vi "main.vi"(8 "Error In":errorcluster, 9 "Simulation Module":bool[](array[boolean]), 10 "Application Path Cluster":T1, 11 "Software Name":string) -> (0 "Error Out":errorcluster)   [LabVIEW 2018]
uses:
  controls/pathCluster.ctl
  UI Module/src/controls/uiData.ctl
  controls/controllerData.ctl
  controls/openModbusConnectionCluster.ctl
  Simulation Module/src/controls/simulationData.ctl
  PLC Module/src/controls/plcData.ctl
  Barcode Scanner Module/src/controls/scanData.ctl
  Barcode Printer Module/src/controls/printData.ctl
  PLC Module/src/controls/plcUDE.ctl
  UI Module/src/controls/uiUDE.ctl
  Simulation Module/src/controls/Simulation UDE.ctl
  <vilib>/event_ctls.llb/usereventprio.ctl
  885446ab-6654-46eb-9afe-71431fbeab30.vi
  367c2bb0-f26a-4887-9fcf-0ea6fc163310.vi
  079b8fb7-678e-4098-9aed-ba415320bfda.vi
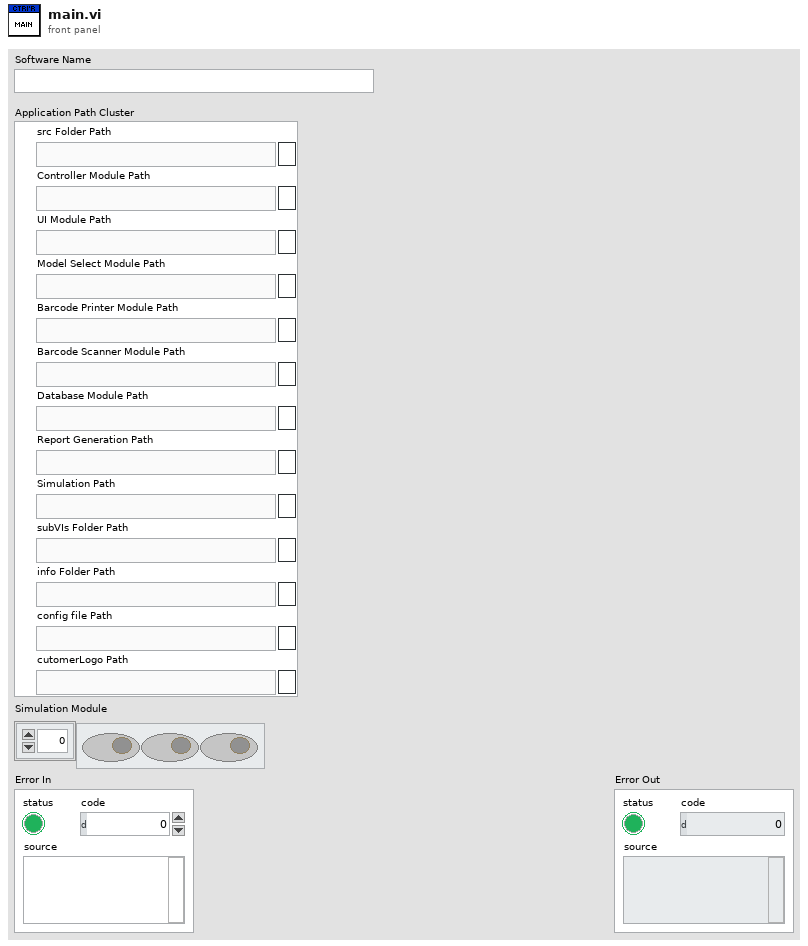
[diagram p1: front panel]
types:
  T1 = typedef "pathCluster.ctl" = cluster{"src Folder Path":path, "Controller Module Path":path, "UI Module Path":path, "Model Select Module Path":path, "Barcode Printer Module Path":path, "Barcode Scanner Module Path":path, "Database Module Path":path, "Report Generation Path":path, "Simulation Path":path, "subVIs Folder Path":path, "info Folder Path":path, "config file Path":path, "cutomerLogo Path":path}
  T2 = enum32{"Invalid", "Standard", "Closed", "Hidden", "Minimized", "Maximized"}
  T3 = enum32{"invalid app kind", "Development System", "Run Time System", "Student Edition", "Embedded LabVIEW", "Evaluation", "Custom"}
  T4 = typedef "plcUDE.ctl" = cluster{"Stop UDE":refnum<user-event>, "PLC UDE":refnum<user-event>}
  T5 = typedef "uiUDE.ctl" = cluster{"UI UDE":refnum<user-event>, "Stop UDE":refnum<user-event>}
  T6 = typedef "Simulation UDE.ctl" = cluster{"Stop UDE":refnum<user-event>, "Simulation Data":refnum<user-event>}
  T7 = typedef "plcData.ctl" = cluster{"IP Address":string, "Timeout":i32, "Port [502]":u16, "isSimulation?":bool, "Model Number":u16}
  T8 = typedef "uiData.ctl" = cluster{"Software Name":string, "UI Module Path":path}
  T9 = typedef "simulationData.ctl" = cluster{"Port [502]":u16, "Model Number":u16}
  T10 = typedef "usereventprio.ctl" = enum32{"high priority", "normal priority"}
  T11 = typedef "openModbusConnectionCluster.ctl" = cluster{"IP Address":string, "Timeout (ms)":i32, "Port (502)":u16}
  T12 = cluster{"Core":cluster{"Current VI Reference":refnum<vi>, "Close Panel on Exit?":bool}, "Software Name":string, "Application Path Cluster":T1, "Simulation Module":bool[], "Open Modbus Connection Cluster":T11, "PLC Data":T7, "Stop UDE":refnum<user-event>, "Simulation UDE":refnum<user-event>, "PLC UDE":refnum<user-event>, "Print Data":refnum<user-event>, "Scan UDE":refnum<user-event>, "Controller UDE":refnum<user-event>, "UI UDE":refnum<user-event>}
  T13 = cluster{"Current VI Reference":refnum<vi>, "Close Panel on Exit?":bool}
  T14 = typedef "scanData.ctl" = cluster{"Scan Button":bool}
  T15 = typedef "printData.ctl" = cluster{"Print Button":bool, "VISA resource name":refnum<visa-resource-name>, "Status?":bool, "Scan?":bool}
  T16 = typedef "controllerData.ctl" = cluster{"Sample":bool}
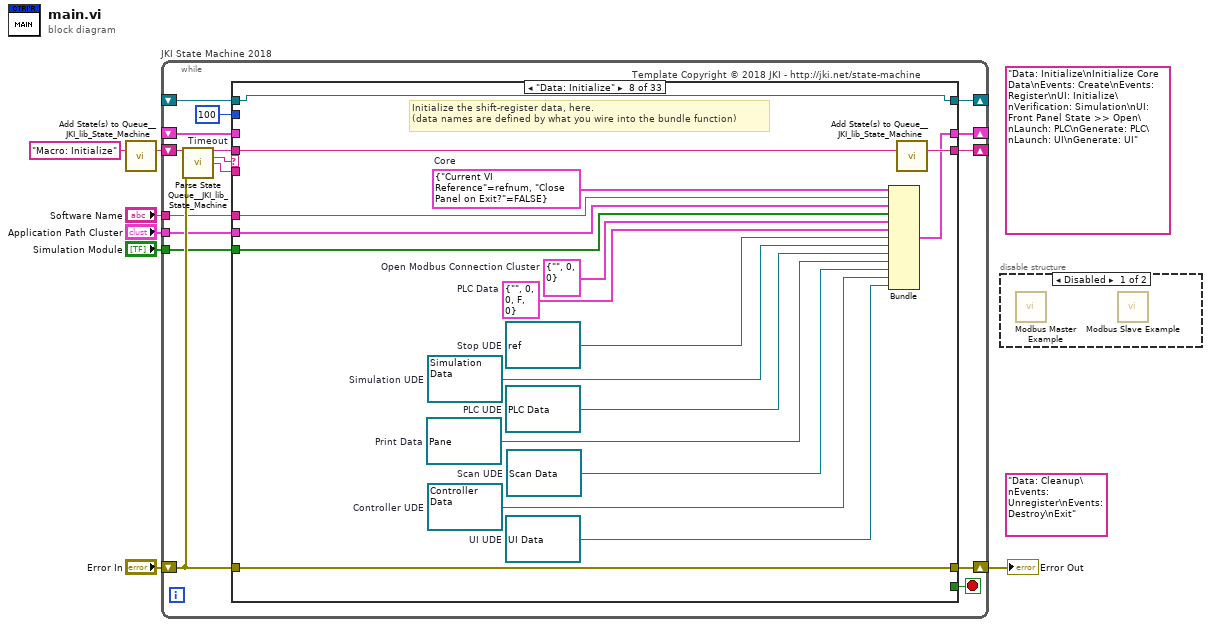
[diagram p0: block diagram]
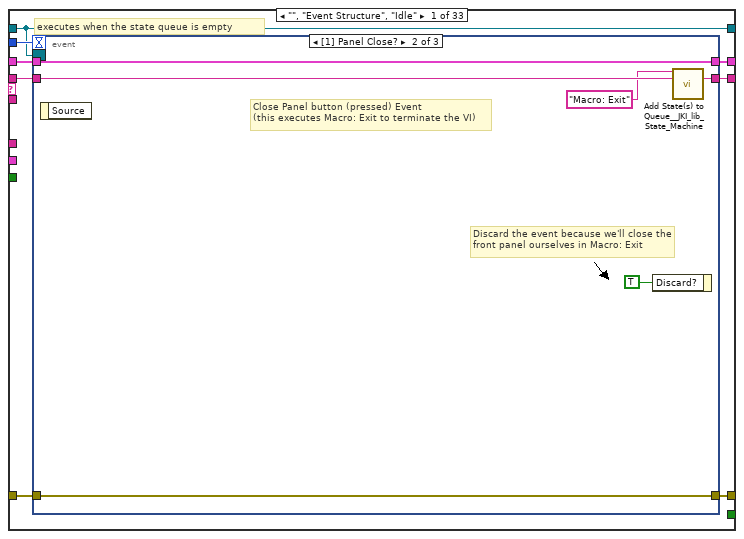
[diagram p3: hidden frame]
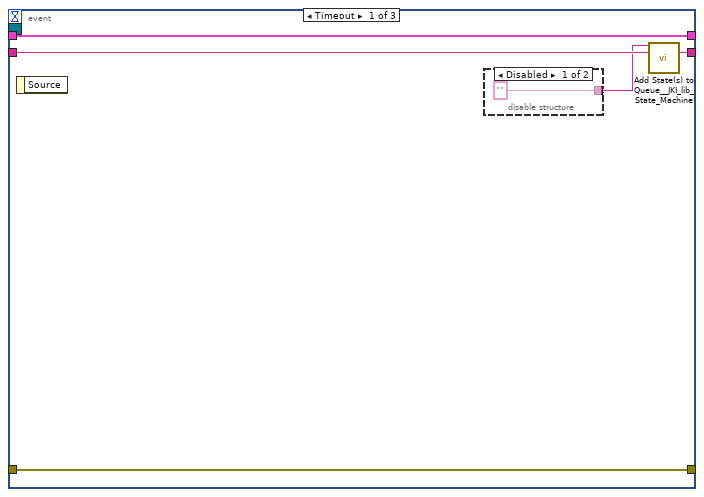
[diagram p4: hidden frame]
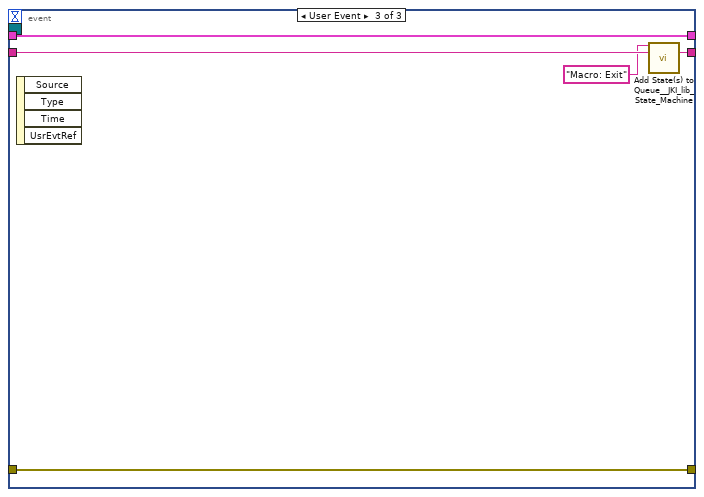
[diagram p6: hidden frame]
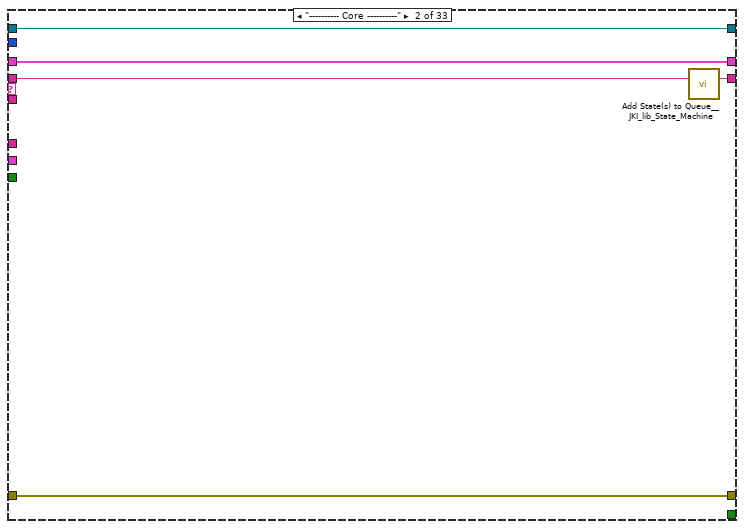
[diagram p7: hidden frame]
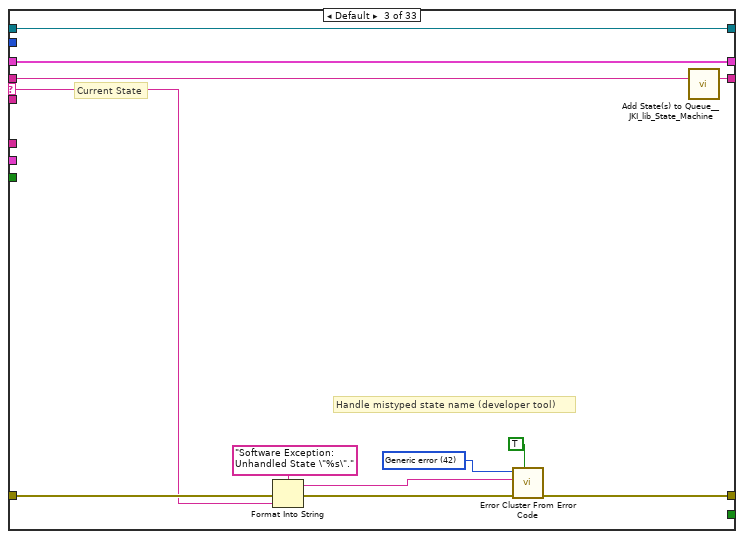
[diagram p8: hidden frame]
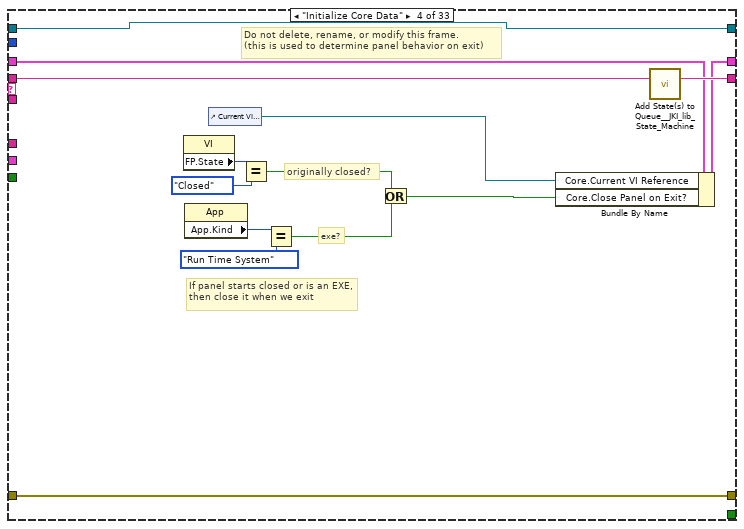
[diagram p9: hidden frame]
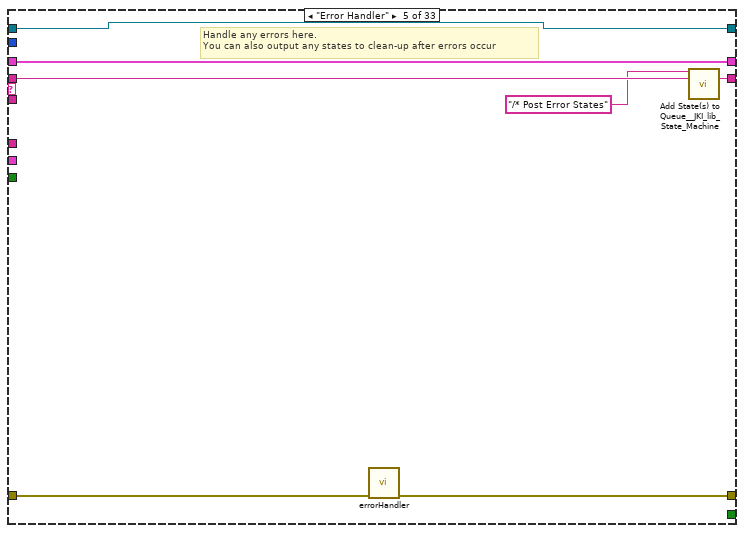
[diagram p10: hidden frame]
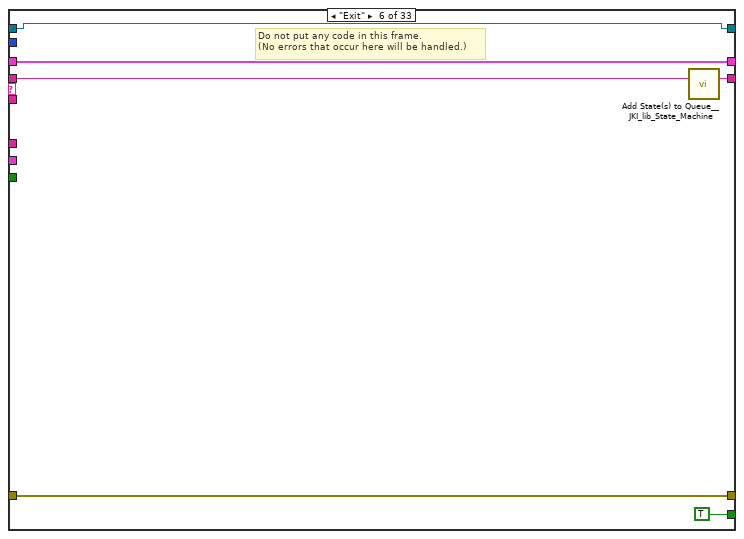
[diagram p11: hidden frame]
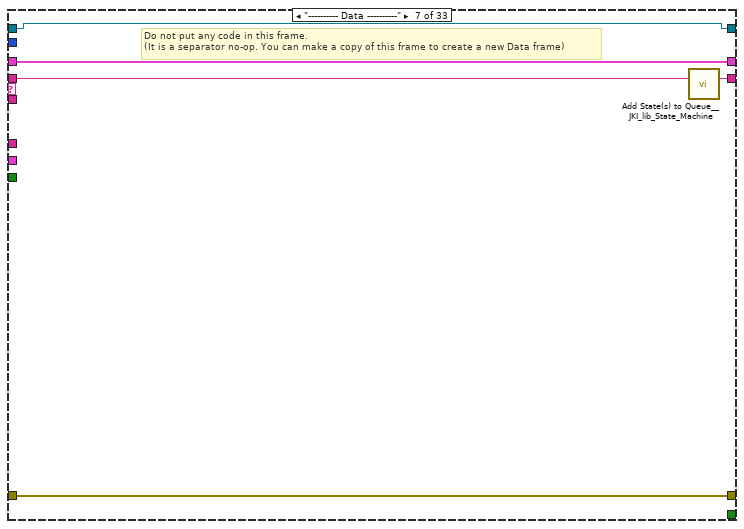
[diagram p12: hidden frame]
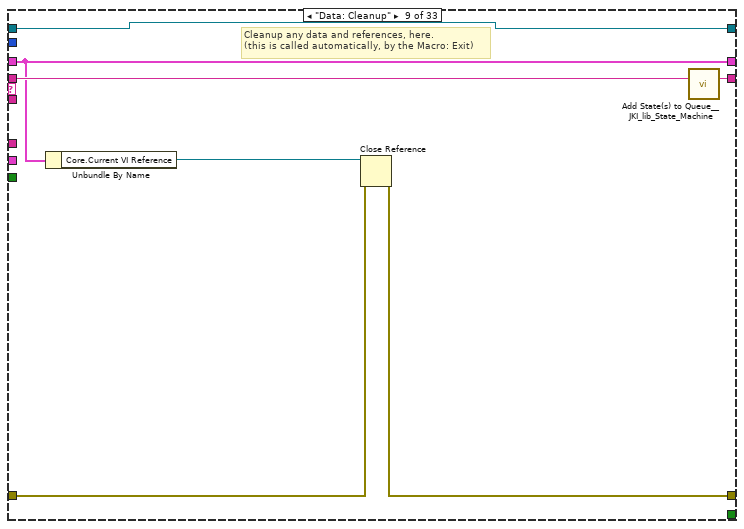
[diagram p13: hidden frame]
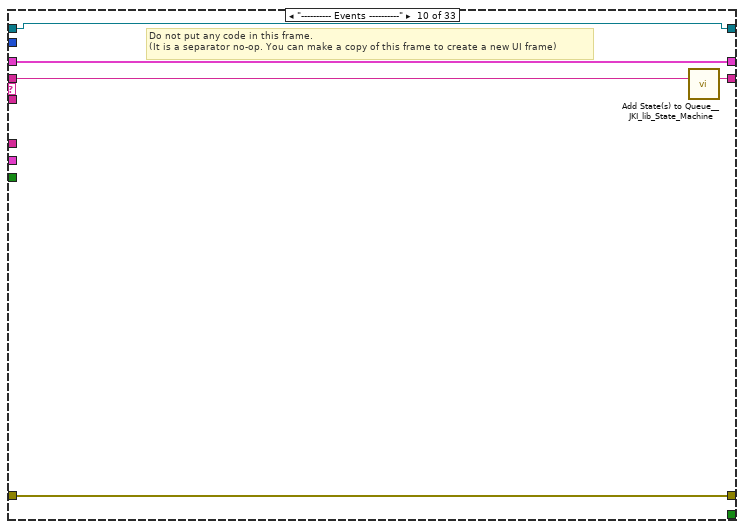
[diagram p14: hidden frame]
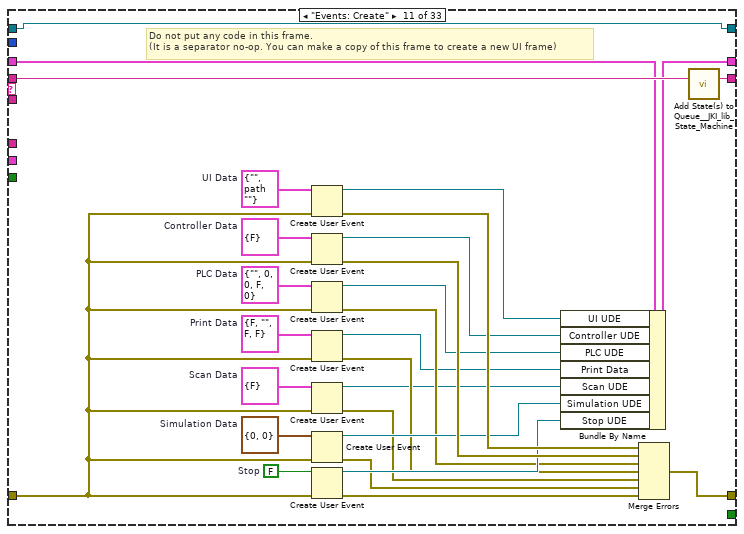
[diagram p15: hidden frame]
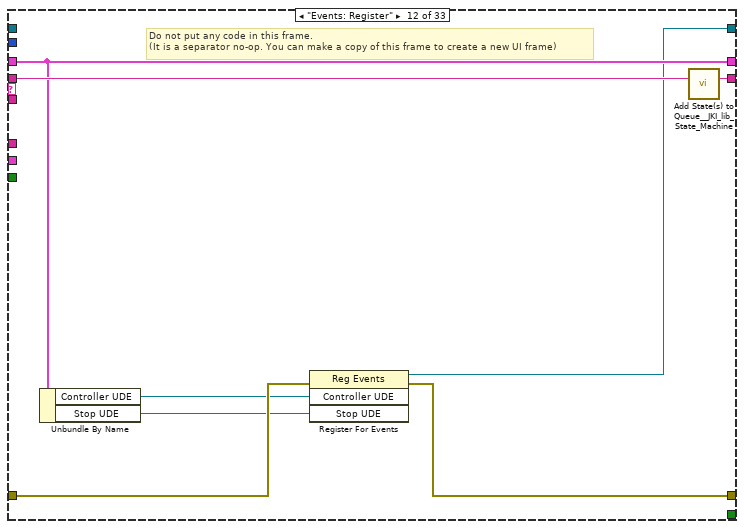
[diagram p16: hidden frame]
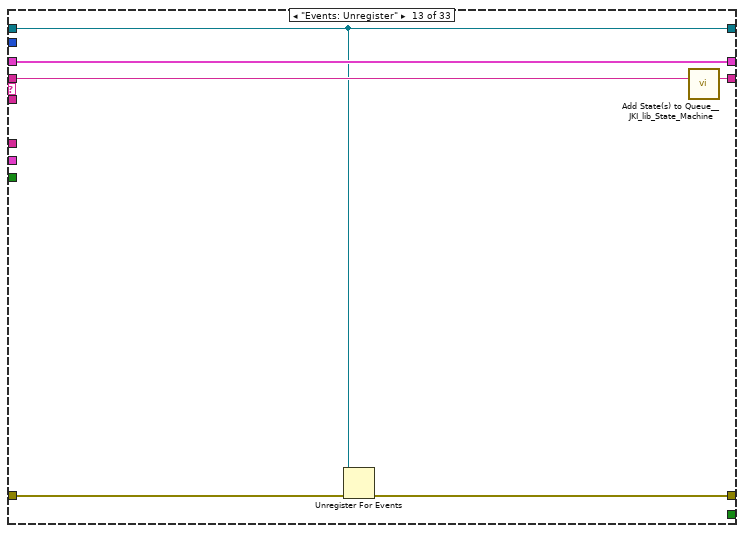
[diagram p17: hidden frame]
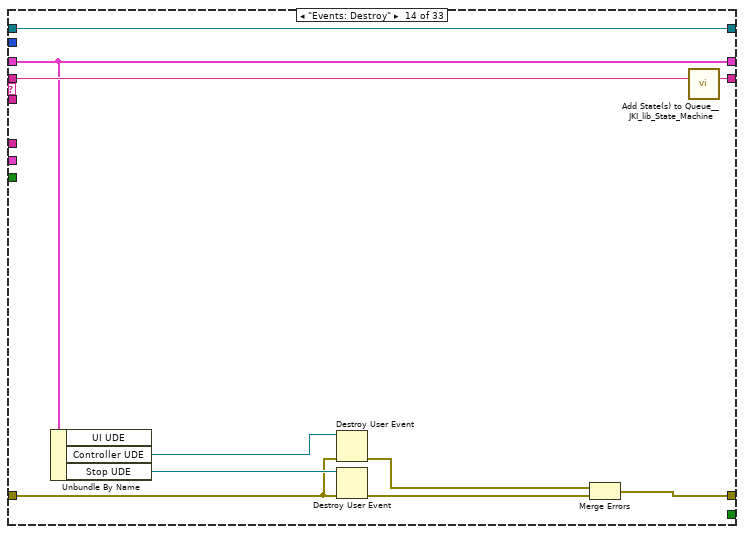
[diagram p18: hidden frame]
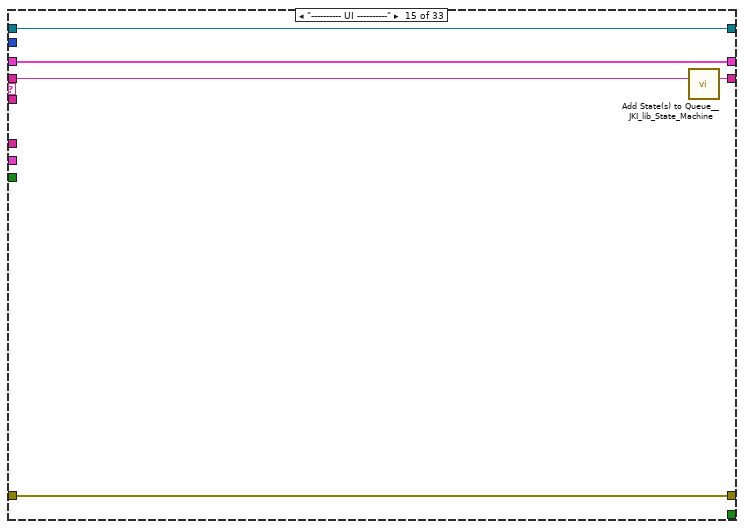
[diagram p19: hidden frame]
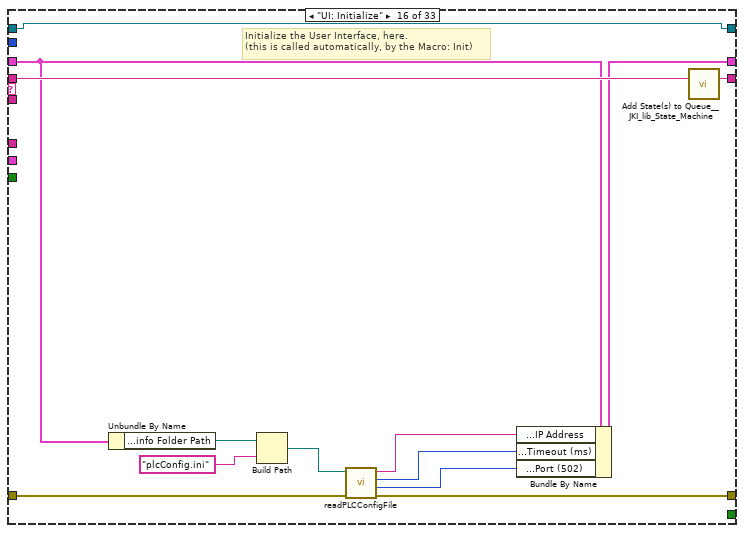
[diagram p20: hidden frame]
diagram:
  (unwired) "Data: Cleanup\nEvents: Unregister\nEvents: Destroy\nExit"
  (unwired) "Data: Initialize\nInitialize Core Data\nEvents: Create\nEvents: Register\nUI: Initialize\nVerification: Simulation\nUI: Front Panel State >> Open\nLaunch: PLC\nGenerate: PLC\nLaunch: UI\nGenerate: UI"
  n1 = call <vilib>:"Add State(s) to Queue__JKI_lib_State_Machine.vi"("State(s) in (\"\")"="Macro: Initialize") -> ("States Out"=w7:string)  [unwired: 14 in]
  n2 = while "JKI State Machine 2018" {
    shift-right: [w16] -> _
    shift-left: _ -> [w15]
    shift-right: [w19] -> w5
    shift-left: "Error In" -> [w13]
    shift-right: [w18] -> _
    shift-left: w7 -> [w20]
    shift-right: [w12] -> _
    shift-left: _ -> [w11]
    tunnel: "Simulation Module" -> [w10]
    tunnel: "Software Name" -> [w9]
    tunnel: "Application Path Cluster" -> [w8]
    stop <- w17 stop-if-true
    w14 = 100  # Timeout
    # "Template Copyright © 2018 JKI - http://jki.net/state-machine"
    n3 = call <vilib>:"Parse State Queue__JKI_lib_State_Machine.vi"("State Queue"=w20, "Error In (no error)"=w13) -> ("Remaining States"=w22:string, "Current State"=w23:string, "Arguments"=w21:string)  [unwired: 11 in]
    n4 = case shown="\"Data: Initialize\"" w23 {
      selector: w23 -> [_ _ w55 _ _ _ _ _ _ _ _ _ _ _ _ _ _ _ _ _ _ _ _ _ _ _ _ _ _ _ _ _ _]
      tunnel: w22 -> [w31 w53 w59 w79 w86 w92 w97 w115 w122 w127 w155 w163 w169 w179 w184 w197 w204 w216 w286 w292 w303 w308 w320 w332 w344 w349 w357 w364 w369 w386 w400 w412 w423]
      tunnel: w21 -> [_ _ _ _ _ _ _ _ _ _ _ _ _ _ _ _ w199 w210 _ _ _ _ _ _ _ _ _ _ _ _ _ _ _]
      tunnel: w15 -> [w29 w50 w57 w72 w84 w90 w94 _ w117 w124 w146 w161 w167 w175 w181 w191 w202 w212 w283 w289 w300 w305 w317 w329 w341 w346 w353 w361 w366 w374 w389 w406 w417]
      tunnel: [w28 w51 w61 w76 w80 w89 w95 w112 w118 w125 w151 w157 w165 w171 w182 w192 w200 w213 w284 w290 w301 w306 w310 w322 w334 w347 w355 w362 w367 w382 w396 w408 w419] -> w19
      tunnel: w13 -> [w27 w51 w60 w76 w81 w89 w95 w112 w119 w125 w128 w160 w166 w172 w182 w193 w201 w214 w284 w290 w301 w306 w316 w325 w339 w347 w355 w362 w367 w383 w397 w409 w420]
      tunnel: [w30 w52 w58 w78 w85 w91 w96 w114 w121 w126 w154 w162 w168 w178 w183 w196 w203 w215 w285 w291 w302 w307 w319 w331 w343 w348 w356 w363 w368 w385 w399 w411 w422] -> w18
      tunnel: [_ _ _ _ _ TRUE _ _ _ _ _ _ _ _ _ _ _ _ _ _ _ _ _ _ _ _ _ _ _ _ _ _ _] -> w17
      tunnel: [w26 w50 w57 w77 w84 w90 w94 w113 w117 w124 w142 w161 w167 w175 w181 w194 w202 w212 w283 w289 w300 w305 w317 w329 w341 w346 w353 w361 w366 w373 w388 w405 w416] -> w16
      tunnel: w14 -> [w25 _ _ _ _ _ _ _ _ _ _ _ _ _ _ _ _ _ _ _ _ _ _ _ _ _ _ _ _ _ _ _ _]
      tunnel: [w24 w49 w54 w66 w82 w87 w93 w107 w116 w123 w141 w156 w164 w177 w180 w195 w198 w209 w282 w287 w293 w304 w318 w330 w342 w345 w354 w360 w365 w384 w398 w410 w421] -> w12
      tunnel: w11 -> [w24 w49 w54 w66 w82 w87 w93 w107 w116 w123 w141 _ w164 w177 w180 w195 w198 w209 w282 w287 w293 w304 w318 w330 w342 w345 w354 w360 w365 w384 w398 w410 w421]
      tunnel: w10 -> [_ _ _ _ _ _ _ w105 _ _ _ _ _ _ _ _ _ _ _ _ _ _ _ _ _ _ _ _ _ _ _ _ _]
      tunnel: w9 -> [_ _ _ _ _ _ _ w104 _ _ _ _ _ _ _ _ _ _ _ _ _ _ _ _ _ _ _ _ _ _ _ _ _]
      tunnel: w8 -> [_ _ _ _ _ _ _ w103 _ _ _ _ _ _ _ _ _ _ _ _ _ _ _ _ _ _ _ _ _ _ _ _ _]
      frame "", "Event Structure", "Idle" {
        # "executes when the state queue is empty"
        n5 = event shown="[1] Panel Close?" {
          selector: w24 -> [_ _ _]
          dyn-events: _ -> [_ _ _]
          timeout: w25 -> [_ _ _]
          tunnel: w31 -> [w36 w43 w46]
          tunnel: [w35 w42 w47] -> w30
          tunnel: w29 -> [w33 w40 w48]
          tunnel: [w34 w41 w44] -> w28
          tunnel: w27 -> [w34 w41 w44]
          tunnel: [w33 w40 w48] -> w26
          event Timeout {
            n6 = event-data() -> ()  [unwired: 1 in, 1 out]
            n7 = disable-structure shown="Disabled" {
              disable-tunnel: ["" _] -> w32
              frame Disabled {
              }
              frame Enabled {
              }
            }
            n8 = call <vilib>:"Add State(s) to Queue__JKI_lib_State_Machine.vi"("State(s) in Front (\"\")"=w32, "State(s) in (\"\")"=w36) -> ("States Out"=w35:string)  [unwired: 13 in]
          }
          event Panel Close? {
            # "Discard the event because we'll close the front panel ourselves in Macro: Exit"
            # "Close Panel button (pressed) Event\n(this executes Macro: Exit to terminate the VI)"
            n9 = event-data() -> ()  [unwired: 1 in, 1 out]
            n10 = event-data("Discard?"=TRUE) -> ()  [unwired: 1 in, 1 out]
            n11 = call <vilib>:"Add State(s) to Queue__JKI_lib_State_Machine.vi"("State(s) in Front (\"\")"="Macro: Exit", "State(s) in (\"\")"=w43) -> ("States Out"=w42:string)  [unwired: 13 in]
          }
          event User Event {
            n12 = event-data() -> ()  [unwired: 1 in, 4 out]
            n13 = call <vilib>:"Add State(s) to Queue__JKI_lib_State_Machine.vi"("State(s) in Front (\"\")"="Macro: Exit" ("State(s) in Front (\"\")"), "State(s) in (\"\")"=w46) -> ("States Out"=w47:string)  [unwired: 13 in]
          }
        }
      }
      frame "---------- Core ----------" {
        n14 = call <vilib>:"Add State(s) to Queue__JKI_lib_State_Machine.vi"("State(s) in (\"\")"=w53) -> ("States Out"=w52:string)  [unwired: 14 in]
      }
      frame Default {
        w64 = 42 items=["No error", "Argument error", "Memory is full", "Out of zone", "End of file", "File already open", "Generic file I/O error", "File not found", "File permission error", "Disk is full", "Duplicate path", "Too many files open", "System feature not enabled", "Resource file not found", "Cannot add resource", "Resource not found", "Image not found", "Image memory error", "Pen does not exist", "Config type invalid", "Config token not found", "Config parse error", "Config memory error", "Bad external code format", "Bad external code offset", "External code not present", "Null window", "Destroy window error", "Null menu", "Print aborted", "Bad print record", "Print driver error", "Windows error during printing", "Memory error during printing", "Print dialog error", "Generic print error", "Invalid device refnum", "Device not found", "Device parameter error", "Device unit error", "Cannot open device", "Device call aborted", "Generic error", "Cancelled by user", "Object ID too low", "Object ID too high", "Object not in heap", "Unknown heap", "Unknown object (invalid DefProc)", "Unknown object (DefProc not in table)", "Message out of range", "Invalid (null) method", "Unknown message", "Manager call not supported", "Bad address", "Network operation in progress", "Network operation timed out", "Connection is busy", "Network attribute not supported", "Network error", "Address in use", "System out of memory", "Connection aborted", "Connection refused", "Not connected", "Already connected", "Connection closed", "Initialization error (interapplication manager)", "Bad occurrence", "Wait on unbound occurrence handler", "Occurrence queue overflow", "Datalog type conflict", "Unused", "Unrecognized type (interapplication manager)", "Memory corrupt", "Failed to make temporary DLL", "Old CIN version", "Drag socket not found", "Failed to load drop-object", "Failed to register OLE object", "Failed to release OLE object", "Format specifier type mismatch", "Unknown format specifier", "Too few format specifiers", "Too many format specifiers", "Scan failed", "Newer CIN version", "Error converting to variant", "Runtime menu error", "Password tampered", "Variant attribute not found", "Incompatible variant data type", "Event data is not available", "Event Store is not present", "Occurrence is not found", "Event Queue is not created", "Event info is not available", "Refnum passed is NULL", "Error retrieving Class GUID", "Error retrieving CoClass GUID", "Error retrieving TypeLib GUID.", "Bad built application magic bytes.", "Specific driver is different from the specific driver associated with the Logical Name.", "There is no session opened to the class driver.", "Max Error", "MAX - Error with config objects", "MAX - Error loading configuration", "MAX - Group not supported"]
        # "Current State"
        # "Handle mistyped state name (developer tool)"
        n15 = Format Into String(format string="Software Exception: Unhandled State \"%s\"." ("message"), error in=w60, w55) -> (resulting string=w63:string, error out=w62:errorcluster)  [unwired: 1 in]
        n16 = call <vilib>:"Error Cluster From Error Code.vi"("show call chain? (False)"=TRUE, "error in (no error)"=w62, "error message (\"\")"=w63, "error code (0)"=w64) -> ("error out"=w61:errorcluster)  [unwired: 5 in]
        n17 = call <vilib>:"Add State(s) to Queue__JKI_lib_State_Machine.vi"("State(s) in (\"\")"=w59) -> ("States Out"=w58:string)  [unwired: 14 in]
      }
      frame "Initialize Core Data" {
        # "Do not delete, rename, or modify this frame.\n(this is used to determine panel behavior on exit)"
        # "originally closed?"
        # "exe?"
        # "If panel starts closed or is an EXE, then close it when we exit"
        n18 = property class="VI"() -> ("FP.State"=w69:T2)  [unwired: 2 in, 2 out]
        n19 = property class="App"() -> ("App.Kind"=w75:T3)  [unwired: 2 in, 2 out]
        n20 = control-ref of="Current VI Reference"() -> (w70:refnum<vi>)
        n21 = Equal?(x=w69, y=T2."Closed" ("Front Panel Window:State")) -> (x = y?=w67:bool)
        n22 = Equal?(x=w75, y=T3."Run Time System" ("Application:Kind")) -> (x = y?=w73:bool)
        n23 = Or(x=w67, y=w73) -> (x .or. y?=w71:bool)
        n24 = Bundle By Name(cluster=w72, "Core.Current VI Reference"=w70, "Core.Close Panel on Exit?"=w71) -> (w77:T12)
        n25 = call <vilib>:"Add State(s) to Queue__JKI_lib_State_Machine.vi"("State(s) in (\"\")"=w79) -> ("States Out"=w78:string)  [unwired: 14 in]
      }
      frame "Error Handler" {
        # "Handle any errors here.\nYou can also output any states to clean-up after errors occur"
        n26 = call "errorHandler.vi"("Error In"=w81) -> ("Error Out"=w80:errorcluster)  [unwired: 10 in]
        n27 = call <vilib>:"Add State(s) to Queue__JKI_lib_State_Machine.vi"("State(s) in Front (\"\")"="/* Post Error States", "State(s) in (\"\")"=w86) -> ("States Out"=w85:string)  [unwired: 13 in]
      }
      frame "Exit" {
        # "Do not put any code in this frame.\n(No errors that occur here will be handled.)"
        n28 = call <vilib>:"Add State(s) to Queue__JKI_lib_State_Machine.vi"("State(s) in (\"\")"=w92) -> ("States Out"=w91:string)  [unwired: 14 in]
      }
      frame "---------- Data ----------" {
        # "Do not put any code in this frame.\n(It is a separator no-op. You can make a copy of this frame to create a new Data frame)"
        n29 = call <vilib>:"Add State(s) to Queue__JKI_lib_State_Machine.vi"("State(s) in (\"\")"=w97) -> ("States Out"=w96:string)  [unwired: 14 in]
      }
      frame "Data: Initialize" {
        w98 = refnum<user-event> refnum  # Print Data
        w99 = refnum<user-event> refnum  # Scan UDE
        w100 = T7 {"IP Address"="", "Timeout"=0, "Port [502]"=0, "isSimulation?"=FALSE, "Model Number"=0}  # PLC Data
        w101 = refnum<user-event> refnum  # PLC UDE
        w102 = refnum<user-event> refnum  # Simulation UDE
        w106 = T11 {"IP Address"="", "Timeout (ms)"=0, "Port (502)"=0}  # Open Modbus Connection Cluster
        w108 = refnum<user-event> refnum  # Stop UDE
        w110 = refnum<user-event> refnum  # Controller UDE
        w109 = refnum<user-event> refnum  # UI UDE
        w111 = T13 {"Current VI Reference"=refnum, "Close Panel on Exit?"=FALSE}  # Core
        # "Initialize the shift-register data, here.\n(data names are defined by what you wire into the bundle function)"
        n30 = Bundle("Core"=w111, "Software Name"=w104, "Application Path Cluster"=w103, "Simulation Module"=w105, "Open Modbus Connection Cluster"=w106, "PLC Data"=w100, "Stop UDE"=w108, "Simulation UDE"=w102, "PLC UDE"=w101, "Print Data"=w98, "Scan UDE"=w99, "Controller UDE"=w110, "UI UDE"=w109) -> (w113:T12)  [unwired: 1 in]
        n31 = call <vilib>:"Add State(s) to Queue__JKI_lib_State_Machine.vi"("State(s) in (\"\")"=w115) -> ("States Out"=w114:string)  [unwired: 14 in]
      }
      frame "Data: Cleanup" {
        # "Cleanup any data and references, here.\n(this is called automatically, by the Macro: Exit)"
        n32 = Unbundle By Name(w117) -> ("Core.Current VI Reference"=w120:refnum<vi>)
        n33 = Close Reference(reference=w120, error in (no error)=w119) -> (error out=w118:errorcluster)
        n34 = call <vilib>:"Add State(s) to Queue__JKI_lib_State_Machine.vi"("State(s) in (\"\")"=w122) -> ("States Out"=w121:string)  [unwired: 14 in]
      }
      frame "---------- Events ----------" {
        # "Do not put any code in this frame.\n(It is a separator no-op. You can make a copy of this frame to create a new UI frame)"
        n35 = call <vilib>:"Add State(s) to Queue__JKI_lib_State_Machine.vi"("State(s) in (\"\")"=w127) -> ("States Out"=w126:string)  [unwired: 14 in]
      }
      frame "Events: Create" {
        w130 = T14 {"Scan Button"=FALSE}  # Scan Data
        w135 = T15 {"Print Button"=FALSE, "VISA resource name"="", "Status?"=FALSE, "Scan?"=FALSE}  # Print Data
        w138 = T7 {"IP Address"="", "Timeout"=0, "Port [502]"=0, "isSimulation?"=FALSE, "Model Number"=0}  # PLC Data
        w140 = T9 {"Port [502]"=0, "Model Number"=0}  # Simulation Data
        w147 = T8 {"Software Name"="", "UI Module Path"=path ""}  # UI Data
        w149 = T16 {"Sample"=FALSE}  # Controller Data
        w152 = FALSE  # Stop
        # "Do not put any code in this frame.\n(It is a separator no-op. You can make a copy of this frame to create a new UI frame)"
        n36 = Create User Event(user event datatype=w147, error in=w128) -> (user event=w143:refnum<user-event>, error out=w148:errorcluster)
        n37 = Create User Event(user event datatype=w149, error in=w128) -> (user event=w144:refnum<user-event>, error out=w150:errorcluster)
        n38 = Create User Event(user event datatype=w138, error in=w128) -> (user event=w136:refnum<user-event>, error out=w137:errorcluster)
        n39 = Create User Event(user event datatype=w135, error in=w128) -> (user event=w134:refnum<user-event>, error out=w133:errorcluster)
        n40 = Create User Event(user event datatype=w130, error in=w128) -> (user event=w131:refnum<user-event>, error out=w132:errorcluster)
        n41 = Create User Event(user event datatype=w140, error in=w128) -> (user event=w139:refnum<user-event>, error out=w129:errorcluster)
        n42 = Create User Event(user event datatype=w152, error in=w128) -> (user event=w145:refnum<user-event>, error out=w153:errorcluster)
        n43 = Bundle By Name(cluster=w146, "UI UDE"=w143, "Controller UDE"=w144, "PLC UDE"=w136, "Print Data"=w134, "Scan UDE"=w131, "Simulation UDE"=w139, "Stop UDE"=w145) -> (w142:T12)
        n44 = Merge Errors(w148, w150, w137, w133, w132, w129, w153) -> (w151:errorcluster)
        n45 = call <vilib>:"Add State(s) to Queue__JKI_lib_State_Machine.vi"("State(s) in (\"\")"=w155) -> ("States Out"=w154:string)  [unwired: 14 in]
      }
      frame "Events: Register" {
        # "Do not put any code in this frame.\n(It is a separator no-op. You can make a copy of this frame to create a new UI frame)"
        n46 = Unbundle By Name(w161) -> ("Controller UDE"=w158:refnum<user-event>, "Stop UDE"=w159:refnum<user-event>)
        n47 = register-events(error in=w160, w158, w159) -> (reference out=w156:refnum<event-registration>, error out=w157:errorcluster)  [unwired: 1 in]
        n48 = call <vilib>:"Add State(s) to Queue__JKI_lib_State_Machine.vi"("State(s) in (\"\")"=w163) -> ("States Out"=w162:string)  [unwired: 14 in]
      }
      frame "Events: Unregister" {
        n49 = Unregister For Events(event registration refnum=w164, error in=w166) -> (error out=w165:errorcluster)
        n50 = call <vilib>:"Add State(s) to Queue__JKI_lib_State_Machine.vi"("State(s) in (\"\")"=w169) -> ("States Out"=w168:string)  [unwired: 14 in]
      }
      frame "Events: Destroy" {
        n51 = Unbundle By Name(w175) -> ("Controller UDE"=w173:refnum<user-event>, "Stop UDE"=w174:refnum<user-event>)  [unwired: 1 out]
        n52 = Destroy User Event(user event=w173, error in=w172) -> (error out=w170:errorcluster)
        n53 = Destroy User Event(user event=w174, error in=w172) -> (error out=w176:errorcluster)
        n54 = Merge Errors(w170, w176) -> (w171:errorcluster)
        n55 = call <vilib>:"Add State(s) to Queue__JKI_lib_State_Machine.vi"("State(s) in (\"\")"=w179) -> ("States Out"=w178:string)  [unwired: 14 in]
      }
      frame "---------- UI ----------" {
        n56 = call <vilib>:"Add State(s) to Queue__JKI_lib_State_Machine.vi"("State(s) in (\"\")"=w184) -> ("States Out"=w183:string)  [unwired: 14 in]
      }
      frame "UI: Initialize" {
        # "Initialize the User Interface, here.\n(this is called automatically, by the Macro: Init)"
        n57 = Unbundle By Name(w191) -> ("Application Path Cluster.info Folder Path"=w190:path)
        n58 = Build Path(base path=w190, name or relative path="plcConfig.ini") -> (appended path=w188:path)
        n59 = call "readPLCConfigFile.vi"("Error In"=w193, "PLC Config File Path"=w188) -> ("Error Out"=w192:errorcluster, "Numeric"=w185:u16, "Port"=w186:i32, "IP Address"=w187:string)  [unwired: 6 in]
        n60 = Bundle By Name(cluster=w191, "Open Modbus Connection Cluster.IP Address"=w187, "Open Modbus Connection Cluster.Timeout (ms)"=w186, "Open Modbus Connection Cluster.Port (502)"=w185) -> (w194:T12)
        n61 = call <vilib>:"Add State(s) to Queue__JKI_lib_State_Machine.vi"("State(s) in (\"\")"=w197) -> ("States Out"=w196:string)  [unwired: 14 in]
      }
      frame "UI: Cursor Set" {
        # "Argument"
        # "Set and Unset Cursor Busy.\n(Usage: \"UI: Cursor Set >> Busy|Idle\")"
        n62 = case shown="\"Idle\", Default" w199 {
          tunnel: w201 -> [w206 w208]
          tunnel: [w205 w207] -> w200
          frame "Idle", Default {
            n63 = call <vilib>:"Unset Busy.vi"("error in (no error)"=w206) -> ("error out"=w205:errorcluster)  [unwired: 10 in]
          }
          frame "Busy" {
            n64 = call <vilib>:"Set Busy.vi"("error in (no error)"=w208) -> ("error out"=w207:errorcluster)  [unwired: 9 in, 1 out]
          }
        }
        n65 = call <vilib>:"Add State(s) to Queue__JKI_lib_State_Machine.vi"("State(s) in (\"\")"=w204) -> ("States Out"=w203:string)  [unwired: 14 in]
      }
      frame "UI: Front Panel State" {
        # "Argument"
        # "Set Front Panel Open or Closed\n(Usage: \"UI: Front Panel State >> Open|Close\")"
        n66 = Unbundle By Name(w212) -> ("Core.Current VI Reference"=w211:refnum<vi>)
        n67 = case shown="\"Close\", \"Closed\"" w210 {
          tunnel: w214 -> [w222 w237 w248 w261 w274]
          tunnel: [w224 w238 w250 w263 w276] -> w213
          tunnel: w211 -> [w223 w235 w249 w262 w275]
          frame "Open", "Standard", Default {
            w217 = T2."Hidden" ("State")
            n68 = property class="VI"(reference=w223, error in=w222) -> (reference out=w220:refnum<vi>, error out=w221:errorcluster, "FP.State"=w219:T2)
            n69 = Not Equal?(x=w219, y=w217) -> (x != y?=w218:bool)
            n70 = case shown="True" w218 {
              tunnel: [w228 w230] -> w224
              tunnel: w221 -> [w227 w230]
              tunnel: w220 -> [w226 _]
              tunnel: w217 -> [w225 _]
              frame True {
                n71 = invoke class="VI" method="FP.Open"(reference=w226, error in=w227, "Activate"=TRUE, "State"=w225) -> (error out=w228:errorcluster)  [unwired: 1 in, 4 out]
              }
              frame False {
              }
            }
          }
          frame "Close", "Closed" {
            n72 = property class="VI"(reference=w235, error in=w237) -> (reference out=w234:refnum<vi>, error out=w236:errorcluster, "FP.State"=w232:T2)
            n73 = Not Equal?(x=w232, y=T2."Closed" ("Front Panel Window:State")) -> (x != y?=w231:bool)
            n74 = case shown="True" w231 {
              tunnel: [w239 w242] -> w238
              tunnel: w236 -> [w239 w241]
              tunnel: w234 -> [_ w240]
              frame False {
              }
              frame True {
                n75 = invoke class="VI" method="FP.Close"(reference=w240, error in=w241) -> (error out=w242:errorcluster)  [unwired: 1 in, 2 out]
              }
            }
          }
          frame "Hidden", "Hide" {
            w243 = T2."Hidden" ("State")
            n76 = property class="VI"(reference=w249, error in=w248) -> (reference out=w246:refnum<vi>, error out=w247:errorcluster, "FP.State"=w245:T2)
            n77 = Not Equal?(x=w245, y=w243) -> (x != y?=w244:bool)
            n78 = case shown="True" w244 {
              tunnel: [w254 w255] -> w250
              tunnel: w247 -> [w253 w255]
              tunnel: w246 -> [w252 _]
              tunnel: w243 -> [w251 _]
              frame True {
                n79 = invoke class="VI" method="FP.Open"(reference=w252, error in=w253, "State"=w251) -> (error out=w254:errorcluster)  [unwired: 2 in, 4 out]
              }
              frame False {
              }
            }
          }
          frame "Minimize", "Minimized" {
            w256 = T2."Minimized" ("State")
            n80 = property class="VI"(reference=w262, error in=w261) -> (reference out=w259:refnum<vi>, error out=w260:errorcluster, "FP.State"=w258:T2)
            n81 = Not Equal?(x=w258, y=w256) -> (x != y?=w257:bool)
            n82 = case shown="True" w257 {
              tunnel: [w267 w268] -> w263
              tunnel: w260 -> [w266 w268]
              tunnel: w259 -> [w265 _]
              tunnel: w256 -> [w264 _]
              frame True {
                n83 = invoke class="VI" method="FP.Open"(reference=w265, error in=w266, "State"=w264) -> (error out=w267:errorcluster)  [unwired: 2 in, 4 out]
              }
              frame False {
              }
            }
          }
          frame "Maximize", "Maximized" {
            w269 = T2."Maximized" ("State")
            n84 = property class="VI"(reference=w275, error in=w274) -> (reference out=w272:refnum<vi>, error out=w273:errorcluster, "FP.State"=w271:T2)
            n85 = Not Equal?(x=w271, y=w269) -> (x != y?=w270:bool)
            n86 = case shown="True" w270 {
              tunnel: [w280 w281] -> w276
              tunnel: w273 -> [w279 w281]
              tunnel: w272 -> [w278 _]
              tunnel: w269 -> [w277 _]
              frame True {
                n87 = invoke class="VI" method="FP.Open"(reference=w278, error in=w279, "State"=w277) -> (error out=w280:errorcluster)  [unwired: 2 in, 4 out]
              }
              frame False {
              }
            }
          }
        }
        n88 = call <vilib>:"Add State(s) to Queue__JKI_lib_State_Machine.vi"("State(s) in (\"\")"=w216) -> ("States Out"=w215:string)  [unwired: 14 in]
      }
      frame "---------- Macro ----------" {
        # "Do not put any code in this frame.\n(It is a separator no-op. You can make a copy of this frame to create a new Macro frame)"
        n89 = call <vilib>:"Add State(s) to Queue__JKI_lib_State_Machine.vi"("State(s) in (\"\")"=w286) -> ("States Out"=w285:string)  [unwired: 14 in]
      }
      frame "Macro: Initialize" {
        # "Initialization Macro\n(This is called once, when the VI starts)"
        n90 = call <vilib>:"Add State(s) to Queue__JKI_lib_State_Machine.vi"("State(s) in Front (\"\")"="Data: Initialize\nInitialize Core Data\nEvents: Create\nEvents: Register\nUI: Initialize\nVerification: Simulation\nUI: Front Panel State >> Open\nLaunch: PLC\nGenerate: PLC\nLaunch: UI\nGenerate: UI", "State(s) in (\"\")"=w292) -> ("States Out"=w291:string)  [unwired: 13 in]
      }
      frame "Macro: Exit" {
        n91 = Unbundle By Name(w300) -> ("Core.Close Panel on Exit?"=w299:bool)
        n92 = Select(t="UI: Front Panel State >> Close", s=w299, f="") -> (s? t:f=w296:string)
        n93 = call <vilib>:"Add State(s) to Queue__JKI_lib_State_Machine.vi"("State(s) in (\"\")"=w296, "State(s) at Back (\"\")"="Data: Cleanup\nEvents: Unregister\nEvents: Destroy\nExit") -> ("States Out"=w294:string)  [unwired: 13 in]
        n94 = call <vilib>:"Add State(s) to Queue__JKI_lib_State_Machine.vi"("State(s) in Front (\"\")"=w294, "State(s) in (\"\")"=w303) -> ("States Out"=w302:string)  [unwired: 13 in]
      }
      frame "---------- Launch ----------" {
        # "Template Separator\n(You can make a copy of, or modify, this frame)"
        n95 = call <vilib>:"Add State(s) to Queue__JKI_lib_State_Machine.vi"("State(s) in (\"\")"=w308) -> ("States Out"=w307:string)  [unwired: 14 in]
      }
      frame "Launch: PLC" {
        # "Template Separator\n(You can make a copy of, or modify, this frame)"
        n96 = Unbundle By Name(w317) -> ("Stop UDE"=w314:refnum<user-event>, "PLC UDE"=w313:refnum<user-event>)
        n97 = Bundle By Name(cluster=T4 {"Stop UDE"=refnum, "PLC UDE"=refnum} ("plcUDE"), "Stop UDE"=w314, "PLC UDE"=w313) -> (w312:T4)
        n98 = call "callPLC.vi"("Error In"=w316, "plcUDE"=w312) -> ("Error Out"=w311:errorcluster)  [unwired: 9 in]
        n99 = call "Stall Data Flow.vim"("value in"=w311, "milliseconds to wait"=u32 100) -> ("value out"=w310:errorcluster)  [unwired: 1 out]
        n100 = call <vilib>:"Add State(s) to Queue__JKI_lib_State_Machine.vi"("State(s) in (\"\")"=w320) -> ("States Out"=w319:string)  [unwired: 14 in]
      }
      frame "Launch: UI" {
        n101 = Unbundle By Name(w329) -> ("UI UDE"=w327:refnum<user-event>, "Stop UDE"=w326:refnum<user-event>)
        n102 = Bundle By Name(cluster=T5 {"UI UDE"=refnum, "Stop UDE"=refnum} ("UDE Data"), "UI UDE"=w327, "Stop UDE"=w326) -> (w324:T5)
        n103 = call "callUI.vi"("Error In"=w325, "UDE Data"=w324) -> ("Error Out"=w323:errorcluster)  [unwired: 9 in]
        n104 = call "Stall Data Flow.vim"("value in"=w323, "milliseconds to wait"=u32 100) -> ("value out"=w322:errorcluster)  [unwired: 1 out]
        n105 = call <vilib>:"Add State(s) to Queue__JKI_lib_State_Machine.vi"("State(s) in (\"\")"=w332) -> ("States Out"=w331:string)  [unwired: 14 in]
      }
      frame "Launch: PLC Slave Sim" {
        n106 = Unbundle By Name(w341) -> ("Simulation UDE"=w340:refnum<user-event>, "Stop UDE"=w336:refnum<user-event>)
        n107 = Bundle By Name(cluster=T6 {"Stop UDE"=refnum, "Simulation Data"=refnum} ("Simulation UDE"), "Simulation Data"=w340, "Stop UDE"=w336) -> (w338:T6)
        n108 = call "callPLCSim.vi"("Error In"=w339, "Simulation UDE"=w338) -> ("Error Out"=w335:errorcluster)  [unwired: 9 in]
        n109 = call "Stall Data Flow.vim"("value in"=w335, "milliseconds to wait"=u32 100) -> ("value out"=w334:errorcluster)  [unwired: 1 out]
        n110 = call <vilib>:"Add State(s) to Queue__JKI_lib_State_Machine.vi"("State(s) in (\"\")"=w344) -> ("States Out"=w343:string)  [unwired: 14 in]
      }
      frame "---------- Verification ----------" {
        # "Template Separator\n(You can make a copy of, or modify, this frame)"
        n111 = call <vilib>:"Add State(s) to Queue__JKI_lib_State_Machine.vi"("State(s) in (\"\")"=w349) -> ("States Out"=w348:string)  [unwired: 14 in]
      }
      frame "Verification: Simulation" {
        # "Template Separator\n(You can make a copy of, or modify, this frame)"
        n112 = Unbundle By Name(w353) -> ("Simulation Module"=w352:bool[])
        n113 = And Array Elements(Boolean array=w352) -> (logical AND=w351:bool)
        n114 = case shown="True" w351 {
          tunnel: ["" "Launch: PLC Slave Sim\nGenerate: PLC Sim" ("State(s) in Front (\"\")")] -> w350
          frame False {
          }
          frame True {
          }
        }
        n115 = call <vilib>:"Add State(s) to Queue__JKI_lib_State_Machine.vi"("State(s) in Front (\"\")"=w350, "State(s) in (\"\")"=w357) -> ("States Out"=w356:string)  [unwired: 13 in]
      }
      frame "---------- PLC ----------" {
        # "Template Separator\n(You can make a copy of, or modify, this frame)"
        n116 = call <vilib>:"Add State(s) to Queue__JKI_lib_State_Machine.vi"("State(s) in (\"\")"=w364) -> ("States Out"=w363:string)  [unwired: 14 in]
      }
      frame "---------- Generate ----------" {
        # "Template Separator\n(You can make a copy of, or modify, this frame)"
        n117 = call <vilib>:"Add State(s) to Queue__JKI_lib_State_Machine.vi"("State(s) in (\"\")"=w369) -> ("States Out"=w368:string)  [unwired: 14 in]
      }
      frame "Generate: PLC" {
        # "Template Separator\n(You can make a copy of, or modify, this frame)"
        n118 = Unbundle By Name(w374) -> ("PLC UDE"=w381:refnum<user-event>, "Open Modbus Connection Cluster"=w378:T11, "Simulation Module"=w371:bool[])
        n119 = Index Array(array=w371) -> (element=w370:bool)  [unwired: 1 in]
        n120 = Unbundle By Name(w378) -> ("IP Address"=w377:string, "Timeout (ms)"=w376:i32, "Port (502)"=w375:u16)
        n121 = Bundle By Name(cluster=T7 {"IP Address"="", "Timeout"=0, "Port [502]"=0, "isSimulation?"=FALSE, "Model Number"=0} ("event data"), "isSimulation?"=w370, "IP Address"=w377, "Timeout"=w376, "Port [502]"=w375) -> (w379:T7)
        n122 = Generate User Event(user event=w381, event data cluster=w379, error in=w383) -> (user event out=w372:refnum<user-event>, error out=w382:errorcluster)  [unwired: 1 in]
        n123 = Bundle By Name(cluster=w374, "PLC UDE"=w372) -> (w373:T12)
        n124 = call <vilib>:"Add State(s) to Queue__JKI_lib_State_Machine.vi"("State(s) in (\"\")"=w386) -> ("States Out"=w385:string)  [unwired: 14 in]
      }
      frame "Generate: UI" {
        # "Template Separator\n(You can make a copy of, or modify, this frame)"
        n125 = Unbundle By Name(w389) -> ("UI UDE"=w395:refnum<user-event>, "Software Name"=w392:string, "Application Path Cluster"=w391:T1)
        n126 = Unbundle By Name(w391) -> ("UI Module Path"=w390:path)
        n127 = Bundle By Name(cluster=T8 {"Software Name"="", "UI Module Path"=path ""} ("event data"), "Software Name"=w392, "UI Module Path"=w390) -> (w393:T8)
        n128 = Generate User Event(user event=w395, event data cluster=w393, error in=w397) -> (user event out=w387:refnum<user-event>, error out=w396:errorcluster)  [unwired: 1 in]
        n129 = Bundle By Name(cluster=w389, "UI UDE"=w387) -> (w388:T12)
        n130 = call <vilib>:"Add State(s) to Queue__JKI_lib_State_Machine.vi"("State(s) in (\"\")"=w400) -> ("States Out"=w399:string)  [unwired: 14 in]
      }
      frame "Generate: PLC Sim" {
        # "Template Separator\n(You can make a copy of, or modify, this frame)"
        n131 = Unbundle By Name(w406) -> ("Simulation UDE"=w407:refnum<user-event>, "Open Modbus Connection Cluster.Port (502)"=w402:u16)
        n132 = Bundle By Name(cluster=T9 {"Port [502]"=0, "Model Number"=0} ("event data"), "Port [502]"=w402) -> (w401:T9)
        n133 = Generate User Event(user event=w407, event data cluster=w401, error in=w409) -> (user event out=w404:refnum<user-event>, error out=w408:errorcluster)  [unwired: 1 in]
        n134 = Bundle By Name(cluster=w406, "Simulation UDE"=w404) -> (w405:T12)
        n135 = call <vilib>:"Add State(s) to Queue__JKI_lib_State_Machine.vi"("State(s) in (\"\")"=w412) -> ("States Out"=w411:string)  [unwired: 14 in]
      }
      frame "Generate: Stop" {
        # "Template Separator\n(You can make a copy of, or modify, this frame)"
        n136 = Unbundle By Name(w417) -> ("Stop UDE"=w418:refnum<user-event>)
        n137 = Generate User Event(priority (normal)=usereventprio."high priority", user event=w418, event data cluster=TRUE, error in=w420) -> (user event out=w415:refnum<user-event>, error out=w419:errorcluster)
        n138 = Bundle By Name(cluster=w417, "Stop UDE"=w415) -> (w416:T12)
        n139 = call <vilib>:"Add State(s) to Queue__JKI_lib_State_Machine.vi"("State(s) in (\"\")"=w423) -> ("States Out"=w422:string)  [unwired: 14 in]
      }
    }
  }
  "Error Out" <- w5
  n140 = disable-structure shown="Disabled" {
    frame Disabled {
      n141 = call <vilib>:"Modbus Master Example.vi"() -> ()  [unwired: 12 in]
      n142 = call <vilib>:"Modbus Slave Example.vi"() -> ()  [unwired: 12 in]
    }
    frame Enabled {
    }
  }
